vi "Publish Data to Array.vi"(11 "Publish Data":T1[](array[typedef])) -> (2 "Status Color":u32[](array[numeric]), 3 "Data[]":string[][](array[string]))   [LabVIEW 2019, in "STS_LTRV.lvlib"]
uses:
  STS_LTRV.lvlib
  TypeDefs/UI Data.ctl
  TypeDefs/Publish Data.ctl
  TypeDefs/NumericLimit Data.ctl
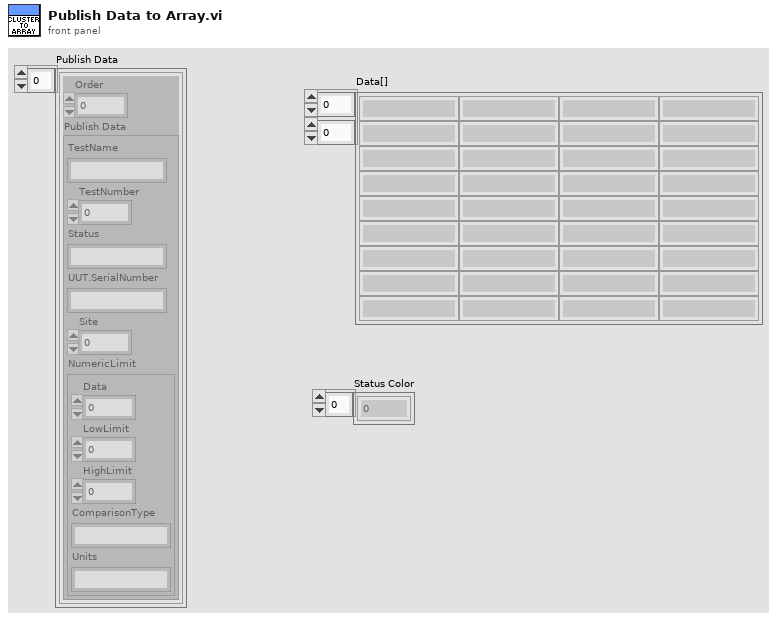
[diagram p1: front panel]
types:
  T1 = typedef "STS_LTRV.lvlib/UI Data.ctl" = cluster{"Order":u64, "Publish Data":T2}
  T2 = typedef "STS_LTRV.lvlib/Publish Data.ctl" = cluster{"TestName":string, "TestNumber":dbl, "Status":string, "UUT.SerialNumber":string, "Site":dbl, "NumericLimit":T3}
  T3 = typedef "STS_LTRV.lvlib/NumericLimit Data.ctl" = cluster{"Data":dbl, "LowLimit":dbl, "HighLimit":dbl, "ComparisonType":string, "Units":string}
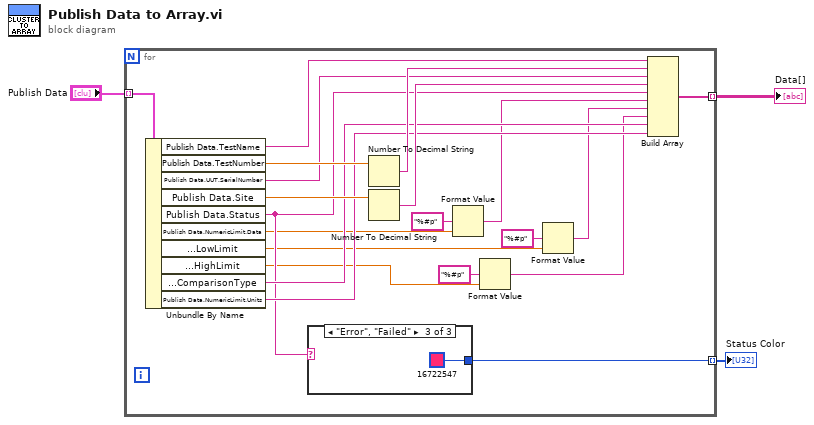
[diagram p0: block diagram]
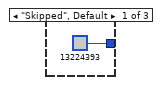
[diagram p2: hidden frame]
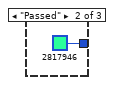
[diagram p3: hidden frame]
diagram:
  n1 = for {
    tunnel: [w16] -> w3 mode=indexing
    tunnel: "Publish Data" -> [w15] mode=indexing
    tunnel: [w13] -> w1 mode=indexing
    n2 = Unbundle By Name(w15) -> ("Publish Data.TestName"=w22:string, "Publish Data.TestNumber"=w24:dbl, "Publish Data.UUT.SerialNumber"=w20:string, "Publish Data.Site"=w23:dbl, "Publish Data.Status"=w14:string, "Publish Data.NumericLimit.Data"=w12:dbl, "Publish Data.NumericLimit.LowLimit"=w8:dbl, "Publish Data.NumericLimit.HighLimit"=w5:dbl, "Publish Data.NumericLimit.ComparisonType"=w18:string, "Publish Data.NumericLimit.Units"=w17:string)
    n3 = case shown="\"Error\", \"Failed\"" w14 {
      tunnel: [u32 13224393 u32 2817946 u32 16722547] -> w13
      frame "Skipped", Default {
      }
      frame "Passed" {
      }
      frame "Error", "Failed" {
      }
    }
    n4 = Number To Decimal String(number=w24) -> (decimal integer string=w21:string)  [unwired: 1 in]
    n5 = Number To Decimal String(number=w23) -> (decimal integer string=w19:string)  [unwired: 1 in]
    n6 = Format Value(format string="%#p", value (0)=w12) -> (output string=w11:string)  [unwired: 1 in]
    n7 = Format Value(format string="%#p", value (0)=w5) -> (output string=w4:string)  [unwired: 1 in]
    n8 = Format Value(format string="%#p", value (0)=w8) -> (output string=w7:string)  [unwired: 1 in]
    n9 = Build Array(w22, w21, w20, w19, w14, w11, w7, w4, w18, w17) -> (w16:string[])
  }
  "Data[]" <- w3
  "Status Color" <- w1
